vi "GitCmd.vi"(4 "Git command":string, 5 "Git exec":string="git") -> (1 "Cmd output":string)   [LabVIEW 2013]
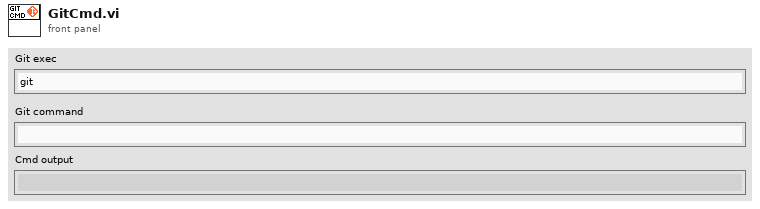
[diagram p1: front panel]
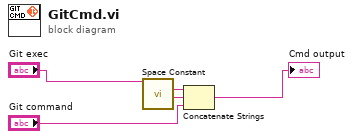
[diagram p0: block diagram]
diagram:
  n1 = call <vilib>:"Space Constant.vi"() -> ("String"=w4:string)
  n2 = Concatenate Strings("Git exec", w4, "Git command") -> (→"Cmd output":string)
